vi "test udp rw.vi"() -> ()   [LabVIEW 2019]
panel:
  out "웨이브폼 차트":dbl(graph)
  in  "대기 시간 (ms)":u32=50
  out "시간 문자열":string="2020-09-25 오후 7:56:52"
  out "port":u16=61556
  out "주소":u32
  out "숫자형":i32=151
  out "데이터 출력":string
  in  "Stop":bool
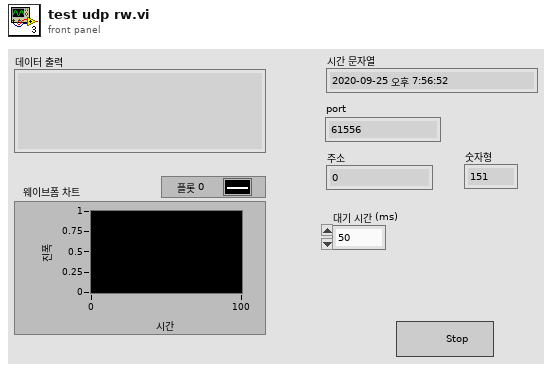
[diagram p1: front panel]
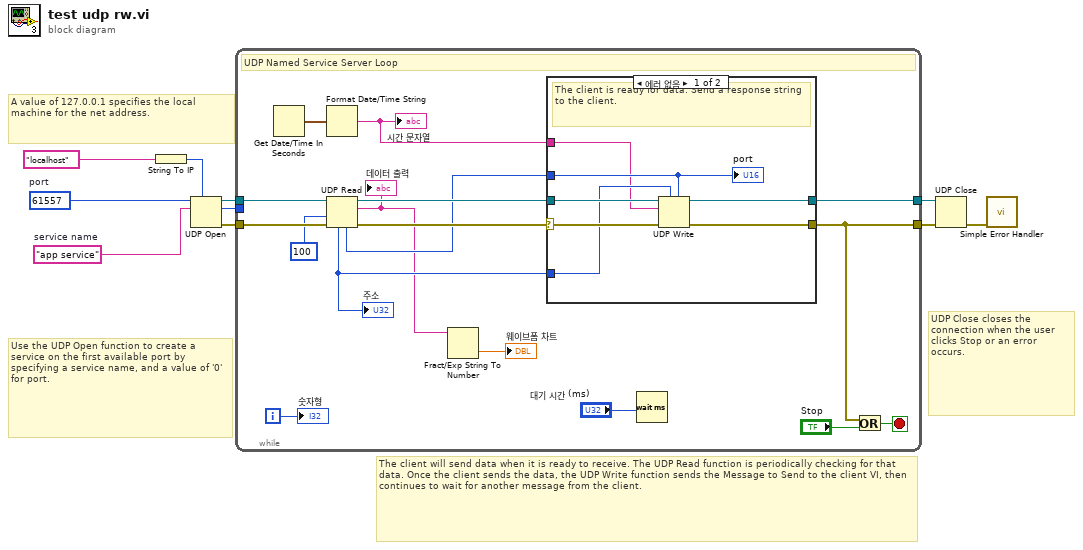
[diagram p0: block diagram]
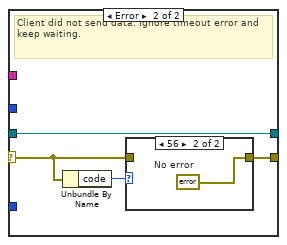
[diagram p2: hidden frame]
diagram:
  w1 = u16 61557  # port
  w10 = "app service"  # service name
  # "UDP Close closes the connection when the user clicks Stop or an error occurs."
  # "A value of 127.0.0.1 specifies the local machine for the net address."
  # "The client will send data when it is ready to receive. The UDP Read function is periodically checking for that data. Once the client sends the data, the UDP Write function sends the Message to Send to the client VI, then continues to wait for another message from the client."
  # "Use the UDP Open function to create a service on the first available port by specifying a service name, and a value of '0' for port."
  n1 = String To IP(1:"localhost") -> (0:w5:u32)
  n2 = UDP Open(7:w5, 10:w10, 11:w1) -> (port=w9:refnum<k16>, 0:w8:errorcluster, 2:w3:u16)  [unwired: 2 in]
  n3 = while {
    tunnel: [w19] -> w6
    tunnel: w9 -> [w27]
    tunnel: w8 -> [w23]
    tunnel: [w24] -> w7
    tunnel: w3 -> [_]
    i -> [w16]
    stop <- w21 stop-if-true
    # "UDP Named Service Server Loop"
    n4 = Get Date/Time In Seconds() -> (seconds since 1Jan1904=w15:timestamp)
    n5 = Format Date/Time String(seconds (now)=w15) -> (date/time string=w14:string)  [unwired: 2 in]
    "시간 문자열" <- w14
    n6 = UDP Read(connection ID=w27, timeout ms (25000)=100, 8:w23) -> (data out=w12:string, error out=w26:errorcluster, 3:w25:refnum<k16>, 4:w22:u16, 6:w17:u32)  [unwired: 1 in]
    "데이터 출력" <- w12
    "주소" <- w17
    n7 = Fract/Exp String To Number(string=w12) -> (number=→"웨이브폼 차트":dbl)  [unwired: 3 in, 1 out]
    n8 = case shown="에러 없음" w26 {
      selector: w26 -> [w34 w37]
      tunnel: w25 -> [w31 w38]
      tunnel: [w33 w35] -> w19
      tunnel: [w32 w38] -> w24
      tunnel: w17 -> [w29 _]
      tunnel: w22 -> [w30 _]
      tunnel: w14 -> [w28 _]
      frame No Error {
        (unwired) TRUE ("초 보이기? (거짓)")
        # "The client is ready for data. Send a response string to the client."
        n9 = UDP Write(address=w29, port or service name=w30, connection ID=w31, data in=w28, 8:w34) -> (error out=w33:errorcluster, 3:w32:refnum<k16>)  [unwired: 1 in]
        "port" <- w30
      }
      frame Error {
        # "Client did not send data. Ignore timeout error and keep waiting."
        n10 = Unbundle By Name(w37) -> ("code"=w36:i32)
        n11 = case shown="56" w36 {
          tunnel: w37 -> [w39 _]
          tunnel: [w39 w40] -> w35
          frame Default {
          }
          frame 56 {
            w40 = errorcluster {"status"=FALSE, "code"=0, "source"=""}  # No error
          }
        }
      }
    }
    n12 = Wait (ms)(milliseconds to wait="대기 시간 (ms)") -> ()  [unwired: 1 out]
    n13 = Or(x=w19, y="Stop") -> (x .or. y?=w21:bool)
    "숫자형" <- w16
  }
  n14 = UDP Close(connection ID=w7, 8:w6) -> (error out=w2:errorcluster)  [unwired: 1 out]
  n15 = call <vilib>:"Simple Error Handler.vi"("error in (no error)"=w2) -> ()  [unwired: 4 in, 5 out]
